vi "12.1 Understanding Clusters.vi"() -> ()   [LabVIEW 2019]
panel:
  in  "Error in":errorcluster
  out "Weather Data output 2":T1
  out "Weather Data output":T1
  out "Temperature Data ºF":T2
  in  "Temperature Data ºC":T2
  in  "Weather Data":T1
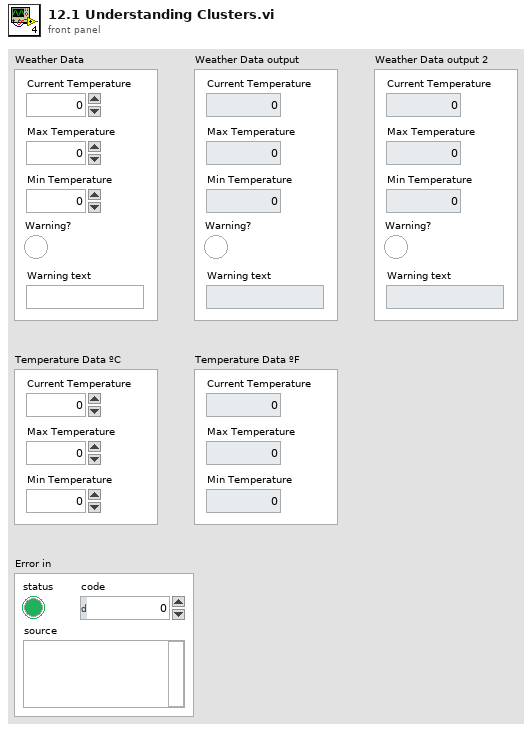
[diagram p1: front panel]
types:
  T1 = cluster{"Current Temperature":dbl, "Max Temperature":dbl, "Min Temperature":dbl, "Warning?":bool, "Warning text":string}
  T2 = cluster{"Max Temperature":dbl, "Current Temperature":dbl, "Min Temperature":dbl}
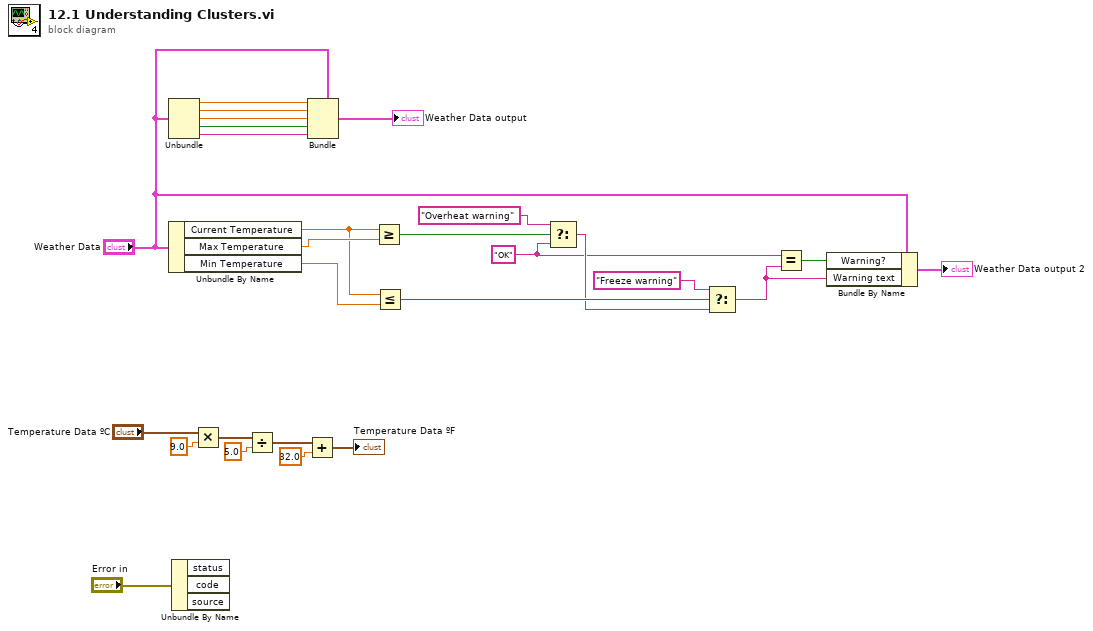
[diagram p0: block diagram]
diagram:
  w5 = "OK"
  n1 = Unbundle "Unbundle"("Weather Data") -> ("Current Temperature"=w20:dbl, "Max Temperature"=w19:dbl, "Min Temperature"=w18:dbl, "Warning?"=w17:bool, "Warning text"=w16:string)
  n2 = Unbundle By Name "Unbundle By Name"("Weather Data") -> ("Current Temperature"=w12:dbl, "Max Temperature"=w13:dbl, "Min Temperature"=w11:dbl)
  n3 = Unbundle By Name("Error in") -> ()  [unwired: 3 out]
  n4 = Multiply(x="Temperature Data ºC", y=9.0) -> (x*y=w27:T2)
  n5 = Divide(x=w27, y=5.0) -> (x/y=w26:T2)
  n6 = Add(x=w26, y=32.0) -> (x+y=→"Temperature Data ºF":T2)
  n7 = Bundle "Bundle"(cluster="Weather Data", "Current Temperature"=w20, "Max Temperature"=w19, "Min Temperature"=w18, "Warning?"=w17, "Warning text"=w16) -> (→"Weather Data output":T1)
  n8 = Greater Or Equal?(x=w12, y=w13) -> (x >= y?=w10:bool)
  n9 = Less Or Equal?(x=w12, y=w11) -> (x <= y?=w8:bool)
  n10 = Select(t="Overheat warning", s=w10, f=w5) -> (s? t:f=w6:string)
  n11 = Select(t="Freeze warning", s=w8, f=w6) -> (s? t:f=w3:string)
  n12 = Equal?(x=w5, y=w3) -> (x = y?=w4:bool)
  n13 = Bundle By Name "Bundle By Name"(cluster="Weather Data", "Warning?"=w4, "Warning text"=w3) -> (→"Weather Data output 2":T1)
